vi "Day 2 Task 1.vi"() -> ()   [LabVIEW 2018]
panel:
  out "Horizontal * vertical (multiplied)":i32
  out "vertical position":i32
  out "horizontal position":i32
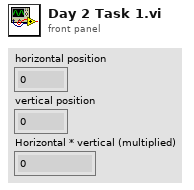
[diagram p1: front panel]
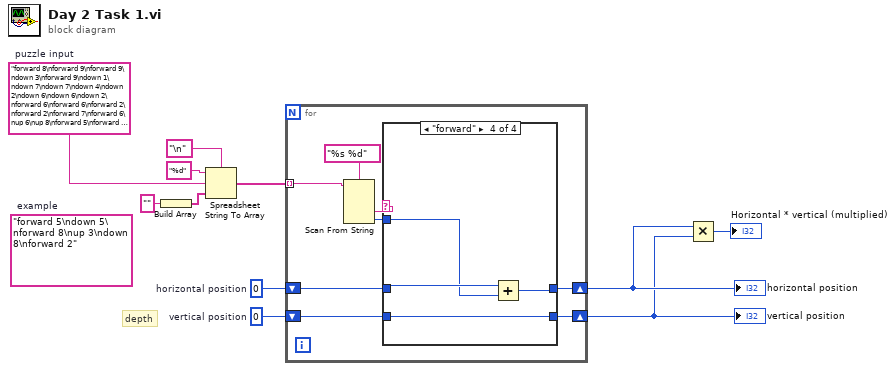
[diagram p0: block diagram]
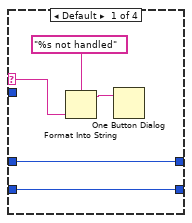
[diagram p2: hidden frame]
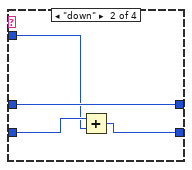
[diagram p3: hidden frame]
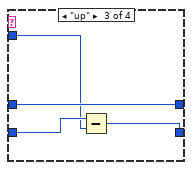
[diagram p4: hidden frame]
diagram:
  w1 = "forward 8\nforward 9\nforward 9\ndown 3\nforward 9\ndown 1\ndown 7\ndown 7\ndown 4\ndown 2\ndown 6\ndown 6\ndown 2\nforward 6\nforward 6\nforward 2\nforward 2\nforward 7\nforward 6\nup 6\nup 8\nforward 5\nforward 4\ndown 6\nforward 7\ndown 5\nforward 5\ndown 8\ndown 8\ndown 7\nforward 4\ndown 2\nforward 7\nup 8\nforward 3\ndown 2\nforward 1\nup 3\nforward 3\nup 1\ndown 3\nup 7\nup 2\ndown 4\ndown 2\nforward 9\nforward 3\ndown 8\nforward 5\nup 9\nup 4\nforward 9\ndown 1\nforward 6\ndown 3\nforward 8\nup 2\nforward 3\nup 7\ndown 4\nforward 2\nforward 7\nforward 3\ndown 1\ndown 3\nup 5\nforward 6\ndown 5\ndown 4\ndown 8\ndown 2\nup 5\nforward 7\nup 8\nforward 2\ndown 5\nforward 3\nup 1\nup 5\ndown 8\ndown 3\nforward 4\nforward 4\nforward 1\nup 8\ndown 9\nforward 7\nforward 9\ndown 5\nup 3\ndown 9\nup 6\nforward 1\nforward 3\nforward 5\ndown 5\nforward 6\ndown 3\ndown 8\nforward 3\nforward 5\nforward 7\nforward 6\ndown 9\ndown 5\ndown 6\ndown 5\ndown 1\ndown 8\nforward 3\ndown 9\ndown 5\ndown 5\nforward 9\nforward 2\ndown 7\nforward 9\nforward 9\nup 1\nforward 3\nup 9\nforward 5\nforward 7\ndown 7\nforward 2\nup 8\nup 6\ndown 7\ndown 3\ndown 5\ndown 2\nforward 6\nforward 6\nup 6\nup 2\nforward 4\nforward 7\nforward 1\ndown 4\nup 8\ndown 3\nup 1\ndown 2\nforward 4\nforward 7\nup 1\ndown 7\nforward 8\nup 2\ndown 8\nup 4\nup 4\nup 2\ndown 8\nup 4\ndown 6\nup 8\ndown 5\nup 5\ndown 8\nforward 9\ndown 1\ndown 5\nforward 3\nforward 3\nup 9\ndown 2\nforward 3\ndown 6\nforward 1\nforward 9\nforward 3\ndown 8\nup 4\ndown 1\ndown 8\nup 1\nforward 2\ndown 7\nup 3\nup 8\ndown 2\nup 6\nforward 6\ndown 9\nforward 4\nforward 7\nup 9\nforward 3\nforward 2\ndown 8\ndown 2\ndown 5\ndown 5\ndown 1\nup 7\ndown 4\nforward 5\ndown 9\ndown 5\ndown 1\ndown 6\nforward 9\ndown 6\nforward 3\ndown 3\nup 6\nforward 2\nforward 6\ndown 2\ndown 9\ndown 6\ndown 1\ndown 7\ndown 6\ndown 6\nup 1\nforward 8\ndown 9\ndown 6\ndown 8\ndown 8\ndown 6\ndown 3\nforward 9\nforward 6\ndown 9\nforward 5\ndown 6\ndown 6\ndown 9\ndown 7\ndown 3\nforward 1\nup 9\nforward 9\ndown 7\nforward 4\ndown 1\nforward 9\nup 9\ndown 7\nforward 5\ndown 3\nup 7\nforward 9\nforward 6\nforward 3\nforward 8\ndown 4\ndown 1\ndown 7\ndown 7\nup 4\ndown 9\nforward 6\nforward 7\ndown 8\nforward 2\nforward 2\nforward 9\nforward 6\nforward 9\nup 6\nup 8\nforward 2\nup 3\nforward 9\nforward 1\ndown 4\nforward 8\ndown 4\nforward 5\nforward 7\nup 2\nforward 5\ndown 4\nforward 3\ndown 5\nforward 9\nup 3\nforward 8\ndown 7\ndown 7\ndown 9\nforward 2\ndown 1\ndown 6\nup 8\ndown 2\ndown 1\nup 3\ndown 3\nforward 2\nforward 6\nup 6\ndown 3\nup 9\nup 3\ndown 8\nup 6\ndown 2\nforward 4\nup 1\ndown 5\ndown 4\nup 9\nup 7\nforward 7\ndown 9\nforward 9\nforward 5\nforward 3\ndown 4\nup 6\nup 7\ndown 7\ndown 6\nup 9\nup 4\ndown 7\nforward 7\nforward 8\ndown 9\nforward 5\nforward 4\ndown 5\nforward 8\nforward 5\nup 3\ndown 9\nforward 1\nforward 2\nup 3\ndown 2\ndown 1\nforward 5\nforward 5\nforward 6\nup 2\nforward 3\ndown 7\ndown 6\nup 3\ndown 4\ndown 4\nforward 5\ndown 3\nup 6\nforward 1\nup 8\nforward 7\nforward 1\nforward 9\ndown 2\nup 8\nup 1\nup 4\nforward 9\nforward 3\nforward 5\ndown 1\nup 9\ndown 1\nforward 3\ndown 6\ndown 8\nup 4\nforward 6\nup 7\ndown 8\nforward 9\nup 2\ndown 7\ndown 1\nforward 9\nup 7\nforward 3\nforward 9\nforward 1\nforward 1\ndown 9\nforward 1\nup 4\ndown 5\nforward 4\ndown 1\nforward 4\nforward 9\nup 4\ndown 3\ndown 6\nup 2\ndown 6\ndown 5\nforward 5\nup 1\nup 9\nforward 8\nup 3\ndown 1\nforward 3\nforward 7\nup 6\nup 3\ndown 6\nforward 7\nup 6\ndown 7\nforward 8\nup 4\ndown 8\nup 9\nup 3\ndown 3\nforward 8\ndown 4\ndown 9\nforward 2\ndown 7\nup 1\nforward 9\nforward 5\nup 8\nforward 9\nforward 4\nforward 9\nforward 7\ndown 4\nup 4\ndown 7\ndown 4\ndown 4\ndown 1\nforward 5\nforward 4\ndown 1\ndown 4\ndown 8\ndown 3\nforward 7\nforward 4\ndown 1\ndown 9\nup 3\nforward 2\ndown 8\ndown 9\ndown 2\ndown 5\nup 9\ndown 9\nup 9\nforward 5\nforward 8\nforward 9\ndown 5\nforward 6\ndown 8\ndown 9\nforward 8\nup 5\nup 9\nup 7\nup 8\nforward 9\nforward 1\nup 6\ndown 8\ndown 8\nforward 1\nup 1\nforward 8\nforward 6\ndown 4\nforward 1\ndown 7\nforward 8\nforward 3\nup 3\ndown 4\ndown 2\nforward 2\nforward 3\nup 4\ndown 3\nforward 2\ndown 8\nforward 7\nup 3\ndown 2\nforward 2\ndown 5\nup 6\nup 6\nforward 4\nup 4\ndown 8\nforward 8\ndown 9\ndown 9\ndown 6\ndown 2\nforward 2\nup 6\nup 5\nforward 3\nforward 3\nup 9\ndown 3\nforward 8\ndown 5\nforward 5\nforward 7\ndown 3\ndown 4\ndown 1\ndown 8\ndown 1\ndown 1\nforward 9\nforward 3\ndown 8\ndown 6\nup 9\nforward 1\nforward 5\nup 9\nup 8\nforward 2\nup 8\ndown 9\nup 2\nforward 5\nforward 1\nforward 8\ndown 3\nforward 4\ndown 5\nup 6\nforward 8\nforward 9\nforward 3\ndown 1\ndown 3\ndown 3\nup 4\nforward 9\ndown 3\ndown 6\nforward 3\nforward 2\ndown 6\ndown 8\nforward 6\nup 8\nup 3\nup 4\nforward 2\nforward 4\nforward 4\nforward 7\ndown 6\nup 8\ndown 3\nforward 8\nforward 4\ndown 7\ndown 5\nforward 6\nforward 4\nforward 6\ndown 3\nforward 3\ndown 1\ndown 7\nforward 3\nforward 2\nforward 7\ndown 5\nup 4\ndown 6\ndown 9\nforward 3\nforward 5\nforward 3\ndown 1\nforward 2\nup 5\nup 6\nforward 2\ndown 4\nforward 3\ndown 4\ndown 1\nforward 8\nup 2\ndown 3\ndown 6\nup 5\nforward 3\nforward 6\ndown 3\nforward 1\ndown 7\nforward 2\nforward 1\nforward 6\nforward 5\nforward 3\ndown 4\ndown 8\nforward 1\nup 2\nup 8\ndown 4\nforward 9\nup 6\nforward 5\nforward 7\ndown 5\nforward 5\ndown 1\nforward 4\nforward 5\nup 2\nforward 5\nup 8\nup 1\nforward 2\ndown 4\ndown 6\nforward 4\ndown 2\ndown 3\nforward 2\nup 3\nup 4\nforward 2\ndown 6\nforward 1\nforward 4\ndown 6\nforward 7\nup 2\nforward 7\nforward 6\nup 2\nforward 8\nforward 4\nforward 9\ndown 1\ndown 8\nforward 3\nforward 2\ndown 8\nup 1\nforward 4\ndown 8\nforward 2\nforward 8\nup 2\ndown 1\nforward 4\nforward 2\nup 4\nup 2\ndown 3\nup 8\nforward 3\nup 8\nforward 9\nup 1\nup 5\ndown 5\ndown 6\nforward 1\nup 5\nup 8\nforward 7\ndown 5\nup 4\nforward 2\nup 4\nup 4\ndown 2\nforward 6\nforward 2\ndown 7\ndown 5\nforward 1\ndown 2\ndown 5\ndown 7\nup 8\ndown 8\nup 5\ndown 1\nforward 5\ndown 2\nforward 5\ndown 1\nup 7\nup 2\nforward 2\nforward 3\nforward 6\nforward 3\ndown 8\nup 8\nforward 8\nforward 1\nforward 7\nup 2\nforward 9\ndown 1\nforward 5\nup 9\nforward 3\nforward 7\nforward 8\nup 1\ndown 3\nforward 5\ndown 2\nforward 6\nforward 3\ndown 9\nup 5\nforward 2\ndown 4\nup 1\nforward 4\nup 4\ndown 8\ndown 8\nforward 3\nforward 8\ndown 7\nup 3\nforward 1\nup 3\nforward 9\nforward 7\nforward 1\ndown 6\nforward 3\ndown 1\ndown 8\nforward 5\nforward 3\nup 6\nforward 5\nforward 4\nforward 3\nforward 9\nforward 8\ndown 6\ndown 2\nforward 7\nforward 6\nup 6\ndown 6\ndown 4\ndown 3\nforward 8\ndown 9\nup 5\nforward 3\nforward 2\ndown 5\nup 4\ndown 6\ndown 3\nforward 9\ndown 2\nforward 9\nforward 8\nup 1\ndown 2\nforward 7\nup 5\nup 6\ndown 8\nup 9\nup 8\nforward 1\nforward 5\ndown 9\nforward 8\ndown 8\nup 1\ndown 7\nforward 7\nup 3\ndown 3\ndown 1\nforward 2\ndown 3\nforward 9\nforward 2\ndown 8\ndown 2\nforward 5\ndown 9\ndown 1\ndown 5\ndown 6\nup 4\nup 3\ndown 1\nup 7\nforward 6\ndown 3\ndown 6\nup 5\nforward 8\nup 8\ndown 1\ndown 2\nup 8\ndown 7\nforward 7\nforward 4\ndown 8\ndown 3\nforward 3\ndown 4\nforward 3\ndown 6\nforward 4\nforward 7\nforward 9\nup 7\nforward 1\ndown 7\ndown 8\ndown 8\nup 6\ndown 3\nforward 5\nforward 5\nforward 9\nforward 4\ndown 4\ndown 8\ndown 7\ndown 1\nforward 2\nforward 4\ndown 3\ndown 6\ndown 7\nforward 5\ndown 8\ndown 1\nforward 4\nforward 3\nforward 1\ndown 6\ndown 7\ndown 1\nforward 6\ndown 4\nup 2\nforward 4\ndown 2\nup 5\ndown 2\ndown 6\nup 7\nforward 4\nforward 7\nforward 9\nup 5\ndown 9\nup 5\nforward 6\ndown 2\nup 8\nup 9\nup 9\nforward 5\ndown 2\nforward 2\ndown 7\nforward 5\nforward 9\nup 8\ndown 8\nforward 1\ndown 2\nup 3\nforward 3\ndown 5\nforward 4\ndown 3\nforward 4\nforward 9\nforward 3\ndown 5\nforward 4\ndown 2\nforward 5\nforward 8\nup 6\nup 2\ndown 3\nforward 6\ndown 5\ndown 4\ndown 4\ndown 4\nup 2\nup 2\nforward 6\nforward 2\nforward 9\ndown 2\ndown 9\ndown 8\nforward 2\ndown 3\nup 3\nforward 5\ndown 4\nup 3\nforward 3\ndown 1\nforward 7\nforward 5\nforward 6\ndown 8\ndown 5\ndown 5\ndown 9\nup 2\nforward 3\ndown 4\ndown 9\nforward 3\nforward 9\nforward 2\nforward 4\nup 6\ndown 6\nup 9\nforward 8\ndown 7\nforward 1\nforward 4\nup 1\nup 2\ndown 9\nforward 6\ndown 6\ndown 1\ndown 4\ndown 7\ndown 6\nforward 5\nup 1\nup 7\ndown 2\ndown 8\ndown 2\ndown 7\ndown 3\nup 9\ndown 7\ndown 5\ndown 6\nforward 9\nup 3\nforward 2\ndown 8\nforward 4\ndown 6\nforward 3\nup 3\ndown 5\nup 4\nforward 6\nforward 7\nforward 9\ndown 3\nforward 7\nforward 3\ndown 4\nup 4\ndown 8\nforward 6\nforward 7\nforward 9\nforward 4\ndown 3\nup 5\ndown 7\ndown 7\nforward 9"  # puzzle input
  w5 = 0  # vertical position
  w6 = 0  # horizontal position
  (unwired) "forward 5\ndown 5\nforward 8\nup 3\ndown 8\nforward 2"  # example
  # "depth"
  n1 = Build Array("") -> (w9:string[])
  n2 = Spreadsheet String To Array(delimiter (Tab)="\n", format string="%d", spreadsheet string=w1, array type (2D Dbl)=w9) -> (array=w7:string[])
  n3 = for {
    tunnel: w7 -> [w17] mode=indexing
    shift-right: [w16] -> w4
    shift-left: w6 -> [w15]
    shift-right: [w13] -> w3
    shift-left: w5 -> [w14]
    n4 = Scan From String(format string="%s %d", input string=w17) -> (output 1=w18:string, output 2=w12:i32)  [unwired: 4 in, 3 out]
    n5 = case shown="\"forward\"" w18 {
      selector: w18 -> [w22 _ _ _]
      tunnel: [w24 w28 w32 w34] -> w16
      tunnel: w15 -> [w24 w28 w32 w35]
      tunnel: w14 -> [w23 w26 w30 w36]
      tunnel: [w23 w27 w31 w36] -> w13
      tunnel: w12 -> [_ w25 w29 w33]
      frame Default {
        n6 = Format Into String(format string="%s not handled", w22) -> (resulting string=w21:string)  [unwired: 2 in, 1 out]
        n7 = One Button Dialog(message=w21) -> ()  [unwired: 1 in, 1 out]
      }
      frame "down" {
        n8 = Add(x=w26, y=w25) -> (x+y=w27:i32)
      }
      frame "up" {
        n9 = Subtract(x=w30, y=w29) -> (x-y=w31:i32)
      }
      frame "forward" {
        n10 = Add(x=w35, y=w33) -> (x+y=w34:i32)
      }
    }
  }
  "horizontal position" <- w4
  "vertical position" <- w3
  n11 = Multiply(x=w4, y=w3) -> (x*y=→"Horizontal * vertical (multiplied)":i32)
